vi "NetComm_ObserveUserProgramStarting.vi"(8 "error in (no error)":errorcluster) -> (0 "error out":errorcluster)   [LabVIEW 2017]
uses:
  FRC_NetworkCommunication.dll
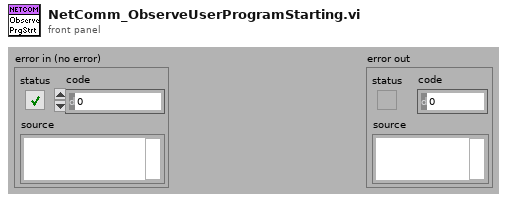
[diagram p1: front panel]
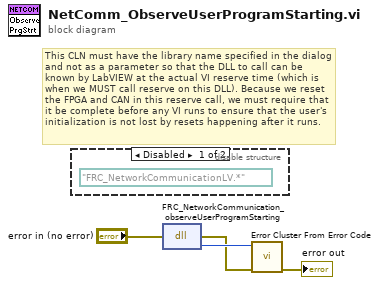
[diagram p0: block diagram]
diagram:
  # "This CLN must have the library name specified in the dialog and not as a parameter so that the DLL to call can be known by LabVIEW at the actual VI reserve time (which is when we MUST call reserve on this DLL). Because we reset the FPGA and CAN in this reserve call, we must require that it be complete before any VI runs to ensure that the user's initialization is not lost by resets happening after it runs."
  n1 = disable-structure shown="Disabled" {
    frame Disabled {
      (unwired) path "FRC_NetworkCommunicationLV.*" ("path in")
    }
    frame Enabled {
    }
  }
  n2 = dll-call lib="FRC_NetworkCommunication.*" fn="FRC_NetworkCommunication_observeUserProgramStarting"(error in="error in (no error)") -> (error out=w3:errorcluster, "return type"=w4:i32)  [unwired: 2 in, 1 out]
  n3 = call <vilib>:"Error Cluster From Error Code.vi"("error in (no error)"=w3, "error code (0)"=w4) -> ("error out"=→"error out":errorcluster)  [unwired: 7 in]
